vi "Destroy LUT Ref.vi"(8 "error in (no error)":errorcluster, 11 "LUT in":refnum<class "LUT.lvclass">) -> (0 "error out":errorcluster)   [LabVIEW 2017, in "LUT.lvlib" / "LUT.lvclass"]
doc: "Destriy the referenc of the look up tabel (LUT)."
uses:
  LUT.lvclass
  LUT.lvclass/LUT.ctl
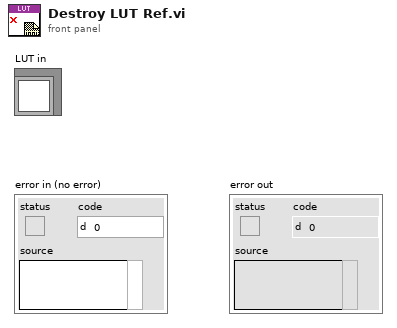
[diagram p1: front panel]
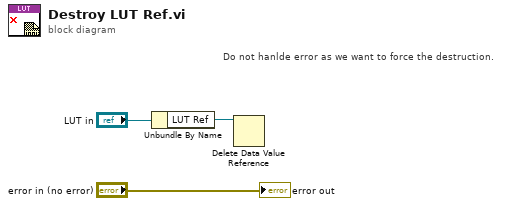
[diagram p0: block diagram]
diagram:
  # "Do not hanlde error as we want to force the destruction."
  n1 = Unbundle By Name("LUT in") -> ("LUT Ref"=w1:refnum<data-value>)
  n2 = Delete Data Value Reference(data value reference=w1) -> ()  [unwired: 1 in, 2 out]
  "error out" <- "error in (no error)"
